vi "Obtain Session.vi"(0 "Filename":string="tg_config.ini", 11 "error in (no error)":errorcluster) -> (4 "Session Handle":T1, 15 "error out":errorcluster)   [LabVIEW 2016, in "_Configurations.lvlib" / "Configurations.lvclass"]
doc: "This function initializes the measurement\n\nPass the function a name to obtain an active measurement handle"
uses:
  Configurations.lvclass
  Typedefs/Session Handle.ctl
  C:/Program Files (x86)/National Instruments/LabVIEW 2016/user.lib/_Session Fwk/Session - Root.lvclass
  Configurations.lvclass/Configurations.ctl
  <userlib>/_Session Fwk/Session - Root.lvclass
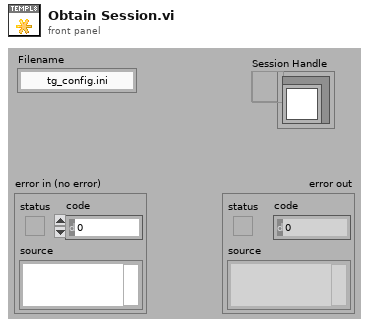
[diagram p1: front panel]
types:
  T1 = typedef "_Configurations.lvlib/Configurations.lvclass/Session Handle.ctl" = refnum<data-value>
  T2 = typedef "Session - Root.lvclass/Session Handle.ctl" = refnum<data-value>
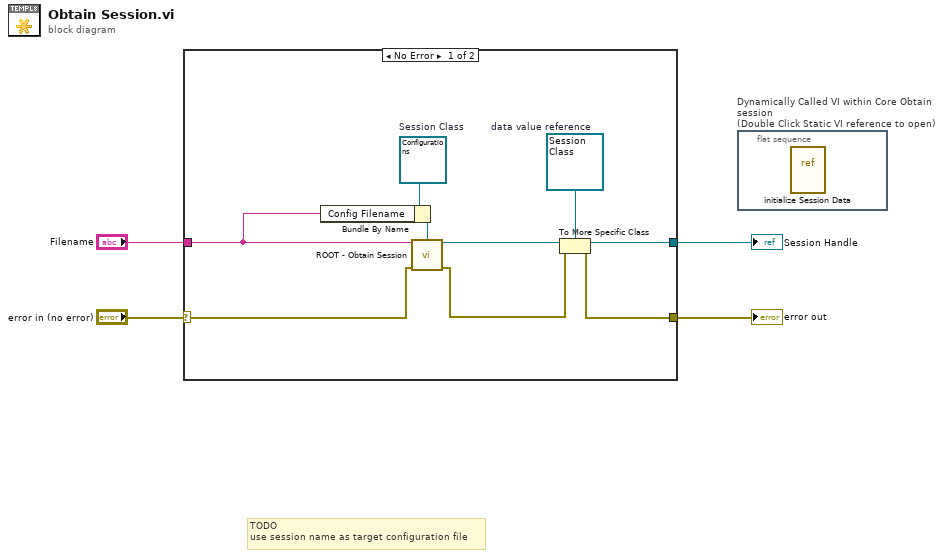
[diagram p0: block diagram]
diagram:
  # "TODO\nuse session name as target configuration file"
  n1 = case shown="No Error" "error in (no error)" {
    selector: "error in (no error)" -> [w6 w14]
    tunnel: [w12 w14] -> w3
    tunnel: [w13 _] -> w1
    tunnel: "Filename" -> [w5 _]
    frame No Error {
      w8 = refnum<data-value> refnum  # data value reference
      w9 = refnum<class "Configurations.lvclass"> refnum  # Session Class
      n2 = Bundle By Name(cluster=w9, "Config Filename"=w5) -> (w10:refnum<class "Configurations.lvclass">)
      n3 = call <userlib>:"ROOT - Obtain Session.vi"("Session Name ()"=w5, "OBJ - Session"=w10, "error in (no error)"=w6) -> ("Session Handle"=w11:T2, "error out"=w7:errorcluster)  [unwired: 10 in, 1 out]
      n4 = To More Specific Class(target class=w8, reference=w11, error in=w7) -> (specific class reference=w13:refnum<data-value>, error out=w12:errorcluster)
    }
    frame Error {
    }
  }
  "error out" <- w3
  "Session Handle" <- w1
  n5 = flat-sequence "Dynamically Called VI within Core Obtain session\n(Double Click Static VI reference to open)" {
    frame #0 {
      n6 = vi-ref "initialize Session Data.vi"() -> ()  [unwired: 1 out]
    }
  }
